vi "test_Find Local Chassis Returns Empty Modules.vi"(8 "error in (no error)":errorcluster, 11 "TestCase in":refnum<class "Scan Engine Scripting API Custom Device Unit Tests.lvclass">) -> (0 "error out":errorcluster, 3 "TestCase out":refnum<class "Scan Engine Scripting API Custom Device Unit Tests.lvclass">)   [LabVIEW 2020, in "Scan Engine Scripting API Custom Device Unit Tests.lvclass"]
uses:
  Scan Engine Scripting API Custom Device Unit Tests.lvclass
  Shared/Type Defs/Local Chassis Settings.ctl
  Scan Engine Scripting API Custom Device Unit Tests.lvclass/Scan Engine Scripting API Custom Device Unit Tests.ctl
  Shared/Type Defs/Main Settings.ctl
  <vilib>/addons/_JKI Toolkits/VI Tester/TestCase.llb/TestCase.lvclass
  Scripting/Scan Engine Scripting.lvlib
  Shared/SEECD Shared.lvlib
  C:/Program Files (x86)/National Instruments/LabVIEW 2020/vi.lib/addons/_JKI Toolkits/VI Tester/TestCase.llb/TestCase.lvclass
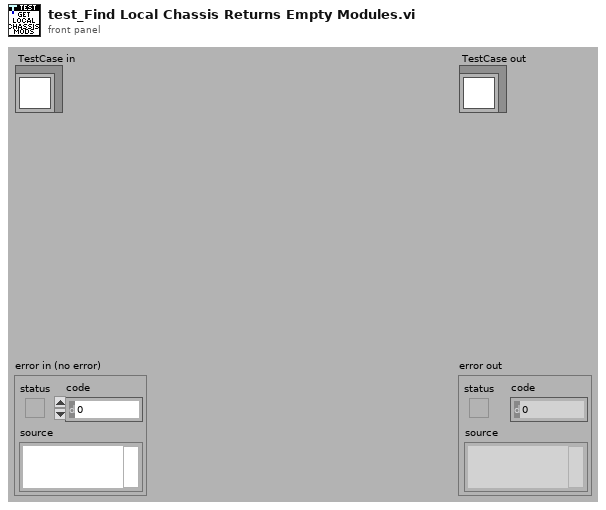
[diagram p1: front panel]
types:
  T1 = typedef "SEECD Shared.lvlib/Local Chassis Settings.ctl" = cluster{"name":string, "number of slots":i32}
  T2 = typedef "SEECD Shared.lvlib/Main Settings.ctl" = cluster{"sync to scan":bool, "scan engine decimation":u16, "delay after FPGA load (s)":u16}
  T3 = typedef "Custom Device API.lvlib/Custom Device Item Ref.ctl" = u64
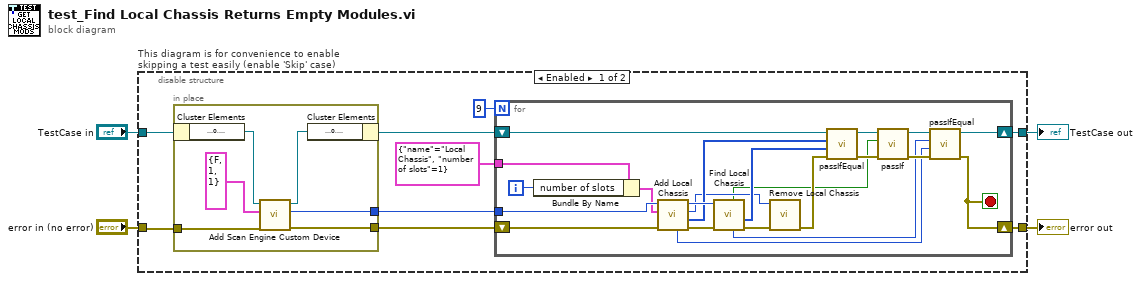
[diagram p0: block diagram]
diagram:
  n1 = disable-structure "This diagram is for convenience to enable skipping a test easily (enable 'Skip' case)" shown="Enabled" {
    disable-tunnel: "TestCase in" -> [w7 w45]
    disable-tunnel: [w8 w43] -> w1
    disable-tunnel: [w13 w44] -> w3
    disable-tunnel: "error in (no error)" -> [w9 w42]
    frame Enabled {
      n2 = in-place {
        in-place-border: [w41] -> w11
        in-place-border: [w40] -> w10
        in-place-border: w9 -> [w38]
        n3 = in-place-cluster #1(w7) -> ("target ref"=w37:refnum<k24>)
        n4 = call "Add Scan Engine Custom Device.vi"("error in"=w38, "settings"=T2 {"sync to scan"=FALSE, "scan engine decimation"=1, "delay after FPGA load (s)"=1}, "target in"=w37) -> ("error out"=w40:errorcluster, "scan engine custom device ref"=w41:T3, "target out"=w36:refnum<k24>)  [unwired: 6 in]
        n5 = in-place-cluster #1("target ref"=w36) -> (w6:refnum<class "Scan Engine Scripting API Custom Device Unit Tests.lvclass">)
      }
      n6 = for {
        N: 9 -> [_]
        tunnel: T1 {"name"="Local Chassis", "number of slots"=1} ("settings") -> [w35]
        tunnel: w11 -> [w34]
        shift-right: [w18] -> w13
        shift-left: w10 -> [w33]
        shift-right: [w16] -> w8
        shift-left: w6 -> [w30]
        i -> [w25]
        stop <- w18 stop-if-true
        n7 = Bundle By Name(cluster=w35, "number of slots"=w25) -> (w26:T1)
        n8 = call "Add Local Chassis.vi"("error in"=w33, "settings"=w26, "scan engine custom device ref in"=w34) -> ("error out"=w31:errorcluster, "slot refs"=w28:T3[], "local chassis ref"=w23:T3, "scan engine custom device ref out"=w32:T3, "user variables ref"=w14:T3)  [unwired: 4 in]
        n9 = call "Find Local Chassis.vi"("error in"=w31, "scan engine custom device ref in"=w32) -> ("error out"=w29:errorcluster, "slots refs"=w27:T3[], "user variables ref"=w15:T3, "found"=w19:bool)  [unwired: 4 in, 2 out]
        n10 = call "Remove Local Chassis.vi"("error in"=w29, "local chassis ref"=w23) -> ("error out"=w24:errorcluster)  [unwired: 9 in]
        n11 = call-dynamic "passIfEqual.vi"("error in (no error)"=w24, "y"=w27, "x"=w28, "TestCase in"=w30) -> ("error out"=w22:errorcluster, "TestCase out"=w20:refnum<class "Scan Engine Scripting API Custom Device Unit Tests.lvclass">)  [unwired: 6 in]
        n12 = call-dynamic "passIf.vi"("error in (no error)"=w22, "pass"=w19, "TestCase in"=w20) -> ("error out"=w21:errorcluster, "TestCase out"=w17:refnum<class "Scan Engine Scripting API Custom Device Unit Tests.lvclass">)  [unwired: 7 in]
        n13 = call-dynamic "passIfEqual.vi"("error in (no error)"=w21, "y"=w14, "x"=w15, "TestCase in"=w17) -> ("error out"=w18:errorcluster, "TestCase out"=w16:refnum<class "Scan Engine Scripting API Custom Device Unit Tests.lvclass">)  [unwired: 6 in]
      }
    }
    frame Disabled {
      # "skip test result while test is under development"
      n14 = call <vilib>:"skip.vi"("error in (no error)"=w42, "TestCase in"=w45) -> ("error out"=w44:errorcluster, "TestCase out"=w43:refnum<class "Scan Engine Scripting API Custom Device Unit Tests.lvclass">)  [unwired: 8 in]
    }
  }
  "error out" <- w3
  "TestCase out" <- w1
